vi "CLD 7 Time Stamp to Initialization String exercise.vi"(8 "Error In":errorcluster) -> (0 "Error Out":errorcluster, 3 "Code String Out":string)   [LabVIEW 2018]
doc: "CLD 7 exercise"
panel:
  out "Ano":string
  out "Mês":string
  out "Dia":string
  out "Dia da semana":string
  out "Segundos":string
  out "Minutos":string
  out "Horas":string
  out "time string":string
  out "date string":string
  # "Troubleshooting Indicators"
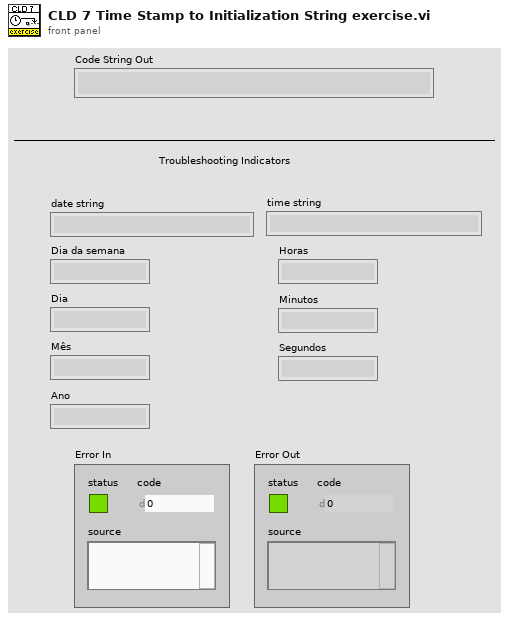
[diagram p1: front panel]
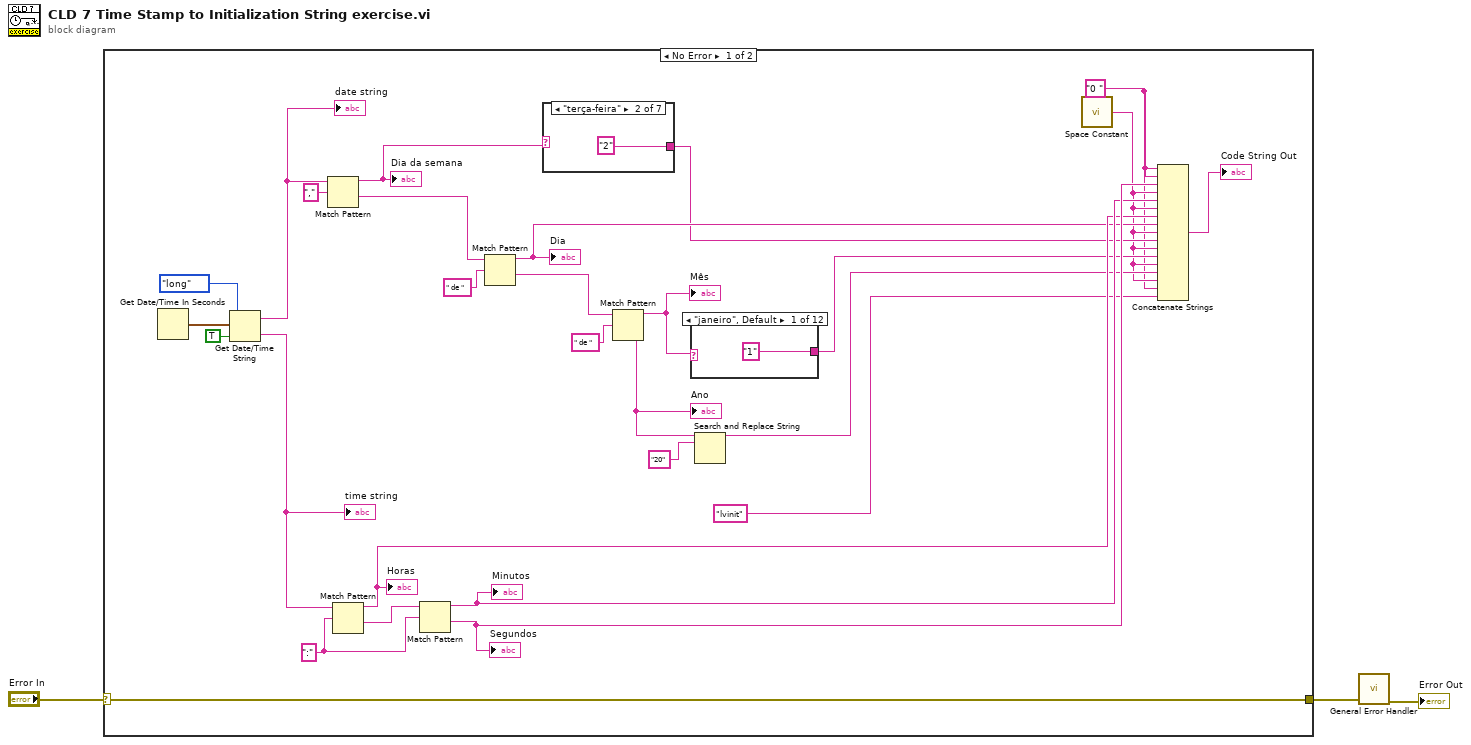
[diagram p0: block diagram]
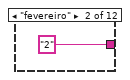
[diagram p2: hidden frame]
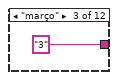
[diagram p3: hidden frame]
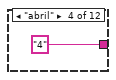
[diagram p4: hidden frame]
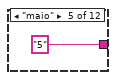
[diagram p5: hidden frame]
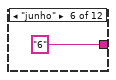
[diagram p6: hidden frame]
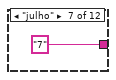
[diagram p7: hidden frame]
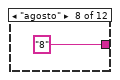
[diagram p8: hidden frame]
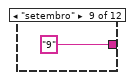
[diagram p9: hidden frame]
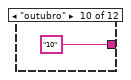
[diagram p10: hidden frame]
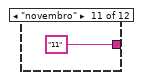
[diagram p11: hidden frame]
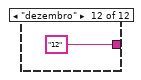
[diagram p12: hidden frame]
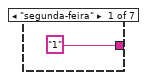
[diagram p13: hidden frame]
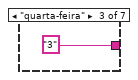
[diagram p14: hidden frame]
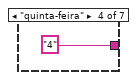
[diagram p15: hidden frame]
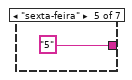
[diagram p16: hidden frame]
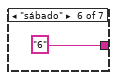
[diagram p17: hidden frame]
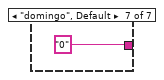
[diagram p18: hidden frame]
diagram:
  n1 = case shown="No Error" "Error In" {
    selector: "Error In" -> [w4 w51]
    tunnel: [w4 w51] -> w2
    frame No Error {
      w25 = ":" ("regular expression")
      w6 = "0 "
      n2 = Get Date/Time In Seconds() -> (seconds since 1Jan1904=w30:timestamp)
      n3 = Get Date/Time String(date format (0)=enum16{"short", "long", "abbreviated"}."long", seconds (now)=w30, want seconds? (F)=TRUE) -> (date string=w21:string, time string=w27:string)
      "date string" <- w21
      "time string" <- w27
      n4 = Match Pattern(string=w21, regular expression=",") -> (before substring=w14:string, after substring=w19:string)  [unwired: 1 in, 2 out]
      "Dia da semana" <- w14
      n5 = Match Pattern(string=w27, regular expression=w25) -> (before substring=w22:string, after substring=w26:string)  [unwired: 1 in, 2 out]
      "Horas" <- w22
      n6 = Match Pattern(string=w26, regular expression=w25) -> (before substring=w23:string, after substring=w24:string)  [unwired: 1 in, 2 out]
      "Minutos" <- w23
      "Segundos" <- w24
      n7 = Match Pattern(string=w19, regular expression=" de ") -> (before substring=w15:string, after substring=w17:string)  [unwired: 1 in, 2 out]
      "Dia" <- w15
      n8 = case shown="\"terça-feira\"" w14 {
        tunnel: ["1" "2" "3" "4" "5" "6" "0"] -> w13
        frame "segunda-feira" {
        }
        frame "terça-feira" {
        }
        frame "quarta-feira" {
        }
        frame "quinta-feira" {
        }
        frame "sexta-feira" {
        }
        frame "sábado" {
        }
        frame "domingo", Default {
        }
      }
      n9 = Match Pattern(string=w17, regular expression=" de ") -> (before substring=w12:string, after substring=w10:string)  [unwired: 1 in, 2 out]
      "Mês" <- w12
      "Ano" <- w10
      n10 = case shown="\"janeiro\", Default" w12 {
        tunnel: ["1" "2" "3" "4" "5" "6" "7" "8" "9" "10" "11" "12"] -> w11
        frame "janeiro", Default {
        }
        frame "fevereiro" {
        }
        frame "março" {
        }
        frame "abril" {
        }
        frame "maio" {
        }
        frame "junho" {
        }
        frame "julho" {
        }
        frame "agosto" {
        }
        frame "setembro" {
        }
        frame "outubro" {
        }
        frame "novembro" {
        }
        frame "dezembro" {
        }
      }
      n11 = Search and Replace String(input string=w10, search string="20") -> (result string=w8:string)  [unwired: 6 in, 3 out]
      n12 = call <vilib>:"Space Constant.vi"() -> ("String"=w7:string)
      n13 = Concatenate Strings(w6, w6, w24, w7, w23, w7, w22, w15, w7, w13, w7, w11, w7, w8, w7, w6, "lvinit") -> (→"Code String Out":string)
    }
    frame Error {
    }
  }
  n14 = call <vilib>:"General Error Handler.vi"("error in (no error)"=w2) -> ("error out"=→"Error Out":errorcluster)  [unwired: 10 in, 4 out]
